vi "Find Quantum Design.vi"(8 "Error In":errorcluster) -> (0 "Error Out":errorcluster, 2 "Names":string[](array[string]), 3 "Recorders List":refnum<class "Instrument Actor.lvclass">[](array[class]))   [LabVIEW 2018, in "Quantum Design.lvclass"]
uses:
  Quantum Design.lvclass
  Instrument Actor/Instrument Actor.lvclass
  C:/github/LabActor/Template Module/Template Module.lvclass
  C:/github/LabActor/Instrument Actor/Instrument Actor.lvclass
  NHMFL_Core/Libraries/Instruments/Quantum Design/Quantum Design Driver/Quantum Design Driver.lvclass
  C:/github/NHMFL_Core/Libraries/Instruments/Instrument Driver/Instrument Driver.lvclass
  Template Module/Template Module.lvclass/Template Module.ctl
  Instrument Actor/Instrument Actor.lvclass/Instrument Actor.ctl
  Template Module/Write Name.vi
  Instrument Actor/Write Instrument driver.vi
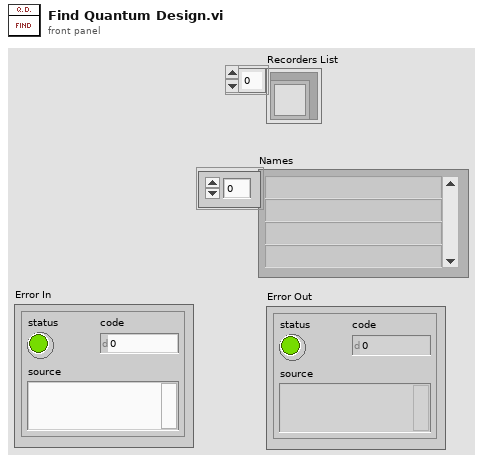
[diagram p1: front panel]
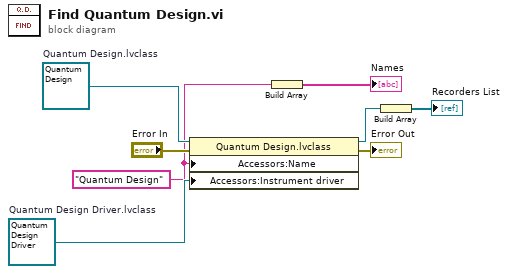
[diagram p0: block diagram]
diagram:
  w4 = refnum<class "Quantum Design Driver.lvclass"> refnum  # Quantum Design Driver.lvclass
  w7 = refnum<class "Quantum Design.lvclass"> refnum  # Quantum Design.lvclass
  w3 = "Quantum Design" ("Name")
  n1 = property class="Quantum Design.lvclass"(reference=w7, error in="Error In", "Accessors:Name"=w3, "Accessors:Instrument driver"=w4) -> (reference out=w2:refnum<class "Quantum Design.lvclass">, error out=→"Error Out":errorcluster)
  n2 = Build Array(w3) -> (→"Names":string[])
  n3 = Build Array(w2) -> (→"Recorders List":refnum<class "Quantum Design.lvclass">[])
